vi "1D Array of VArrays to MultiD Array.vi"(8 "error in (no error)":errorcluster, 10 "Array of VArrays":variant[](array[variant])) -> (0 "error out":errorcluster, 2 "MultiD Array":variant)   [LabVIEW 2013, in "JKI JSON Serialization.lvlib" / "JSON Deserializer.lvclass"]
uses:
  JSON Deserializer.lvclass
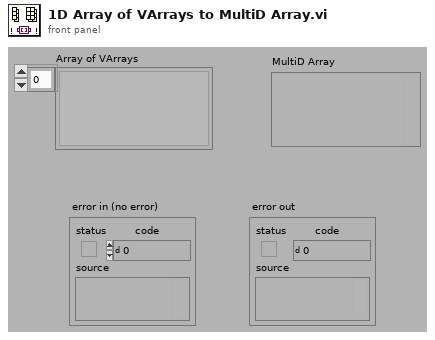
[diagram p1: front panel]
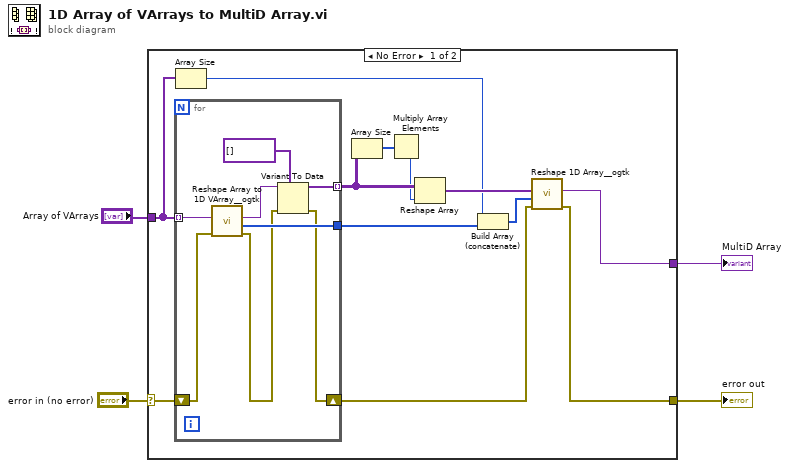
[diagram p0: block diagram]
diagram:
  n1 = case shown="No Error" "error in (no error)" {
    selector: "error in (no error)" -> [w16 w25]
    tunnel: [w9 w25] -> w4
    tunnel: [w5 _] -> w1
    tunnel: "Array of VArrays" -> [w15 _]
    frame No Error {
      n2 = for {
        tunnel: w15 -> [w24] mode=indexing
        shift-right: [w19] -> w10
        shift-left: w16 -> [w23]
        tunnel: [w22] -> w6
        tunnel: [w17] -> w13 mode=indexing
        n3 = call <userlib>:"Reshape Array to 1D VArray__ogtk.vi"("error in (no error)"=w23, "MultiD Array"=w24) -> ("error out"=w20:errorcluster, "Size(s)"=w22:u32[], "1D VArray"=w21:variant)  [unwired: 7 in]
        n4 = Variant To Data(error in=w20, type=variant[] [], Variant=w21) -> (data=w17:variant[], error out=w19:errorcluster)
      }
      n5 = Array Size(array=w15) -> (size(s)=w8:i32)
      n6 = Array Size(array=w13) -> (size(s)=w14:i32[])
      n7 = Multiply Array Elements(1:w14) -> (0:w12:i32)
      n8 = Reshape Array(w13, w12) -> (w11:variant[])
      n9 = Build Array (concatenate)(w8, w6) -> (w7:u32[])
      n10 = call <userlib>:"Reshape 1D Array__ogtk.vi"("error in (no error)"=w10, "Size(s)"=w7, "1D Array"=w11) -> ("error out"=w9:errorcluster, "Reshaped VArray"=w5:variant)  [unwired: 7 in]
    }
    frame Error {
    }
  }
  "error out" <- w4
  "MultiD Array" <- w1
